vi "Format Timestamp To T-SQL Datetime2.vi"(11 "Time":timestamp) -> (3 "datetime2":string)   [LabVIEW 2015, in "Utility.lvlib"]
uses:
  Utility.lvlib
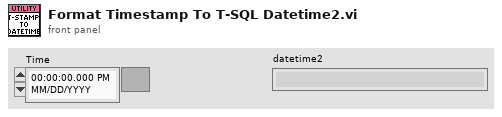
[diagram p1: front panel]
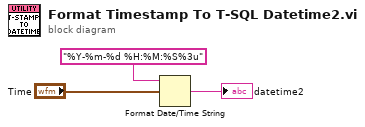
[diagram p0: block diagram]
diagram:
  n1 = Format Date/Time String(time format string (%c)="%Y-%m-%d %H:%M:%S%3u", seconds (now)="Time") -> (date/time string=→"datetime2":string)  [unwired: 1 in]
